vi "数据截取整合.vi"(0 "Input Data":string, 1 "正则表达式":string="[|]", 3 "起始元素":string="ST") -> (6 "整理后的数据":string[](array[string]))   [LabVIEW 2011]
panel:
  out "数组":string[](array[string])
  out "元素索引":i32
  out "匹配后偏移量":i32
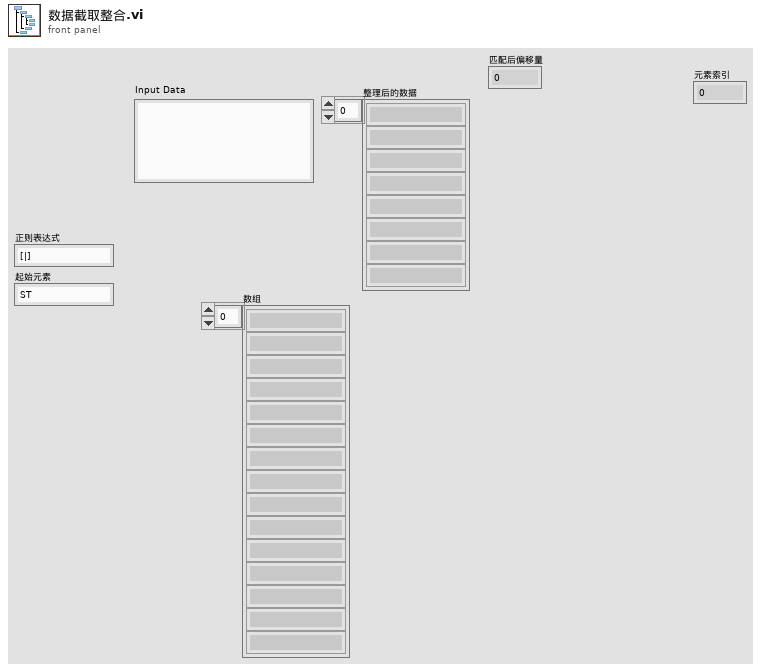
[diagram p1: front panel]
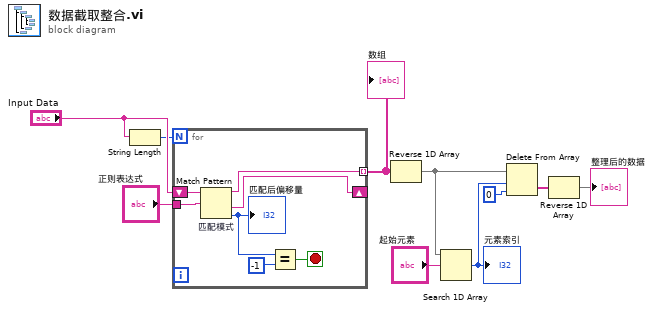
[diagram p0: block diagram]
diagram:
  n1 = String Length(string="Input Data") -> (length=w9:i32)
  n2 = for {
    N: w9 -> [_]
    shift-right: [w16] -> _
    shift-left: "Input Data" -> [w17]
    tunnel: [w15] -> w8 mode=indexing
    tunnel: "正则表达式" -> [w11]
    stop <- w12 stop-if-true
    n3 = Match Pattern "匹配模式"(string=w17, regular expression=w11) -> (before substring=w15:string, after substring=w16:string, offset past match=w14:i32)  [unwired: 1 in, 1 out]
    "匹配后偏移量" <- w14
    n4 = Equal?(x=w14, y=-1) -> (x = y?=w12:bool)
  }
  "数组" <- w8
  n5 = Reverse 1D Array(array=w8) -> (reversed array=w6:string[])
  n6 = Search 1D Array(1D array=w6, element="起始元素") -> (index of element=w5:i32)  [unwired: 1 in]
  "元素索引" <- w5
  n7 = Delete From Array(array=w6, length=w5, index=0 ("索引")) -> (deleted portion=w2:string[])  [unwired: 1 out]
  n8 = Reverse 1D Array(array=w2) -> (reversed array=→"整理后的数据":string[])
